vi "Go to field based on control voltage.vi"(8 "error in":errorcluster, 10 "Control Voltage":dbl min=-9.0 max=9.0 format="%0.2f", 11 "task in":refnum<k21>) -> (0 "error out":errorcluster, 3 "task out":refnum<k21>)   [LabVIEW 2009, in "Varian.lvlib"]
doc: "Writes a control voltage to Varian Magnet through DAQ ao0 channel.\n\nCoerces values to between 9 and -3 V."
uses:
  Varian.lvlib
  <vilib>/DAQmx/write.llb/DAQmx Write (Analog DBL 1Chan 1Samp).vi
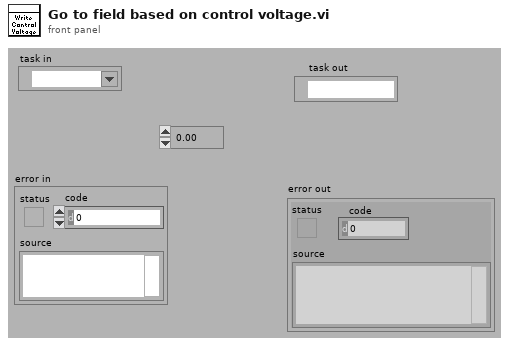
[diagram p1: front panel]
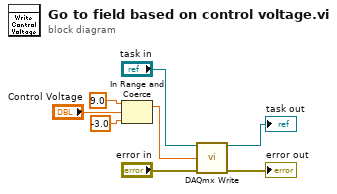
[diagram p0: block diagram]
diagram:
  n1 = In Range and Coerce(upper limit=9.0, x="Control Voltage", lower limit=-3.0) -> (coerced(x)=w6:dbl)  [unwired: 1 out]
  n2 = call-poly <vilib>:"DAQmx Write.vi"("task/channels in"="task in", "data"=w6, "error in"="error in") -> ("task out"=→"task out":refnum<k21>, "error out"=→"error out":errorcluster)  [unwired: 1 in, 10 out]
